vi "Parse Single Measurement.vi"(9 "Offset":i32, 10 "Measurement String":string) -> (1 "Measurement Metadata":T1, 2 "Measurement":dbl, 4 "Offset Past Token":i32)   [LabVIEW 2011, in "Keithley 2182.lvlib"]
doc: "Parses a single measurement into a numerical value and its corresponding metadata.\n\nAssumes all metadata is included in string, which includes:\n\n1. Reading\n2. Unit\n3. Channel\n\n[Mantissa][Exponent][Units], [Channel][Channel Units]\n\ne.g.\n-1.23456789E00VDC, 01INTCHAN"
uses:
  Keithley 2182.lvlib
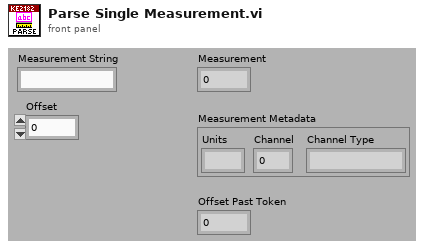
[diagram p1: front panel]
types:
  T1 = cluster{"Units":string, "Channel":i32, "Channel Type":string}
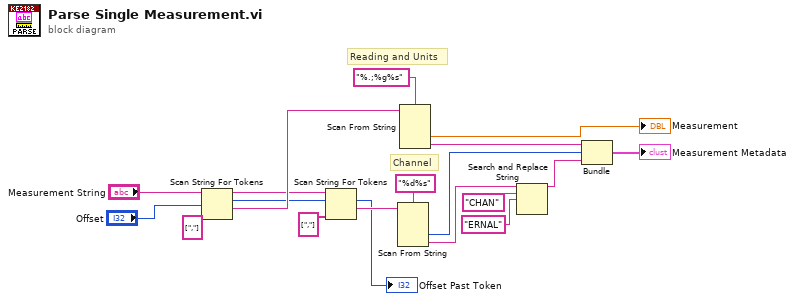
[diagram p0: block diagram]
diagram:
  # "Channel"
  # "Reading and Units"
  n1 = Scan String For Tokens(6:string[] [","] ("delimiters (\\s,\\t,\\r,\\n)"), 8:"Offset", 9:"Measurement String") -> (1:w17:string, 2:w14:i32, 3:w16:string)  [unwired: 3 in, 1 out]
  n2 = Scan String For Tokens(6:string[] [","] ("delimiters (\\s,\\t,\\r,\\n)"), 8:w14, 9:w16) -> (1:w12:string, 2:→"Offset Past Token":i32)  [unwired: 3 in, 2 out]
  n3 = Scan From String(format string="%d%s", input string=w12) -> (output 1=w11:i32, output 2=w10:string)  [unwired: 4 in, 3 out]
  n4 = Scan From String(format string="%.;%g%s", input string=w17) -> (output 1=→"Measurement":dbl, output 2=w13:string)  [unwired: 4 in, 3 out]
  n5 = Search and Replace String(input string=w10, search string="CHAN", replace string="ERNAL" ("replace string (\"\")")) -> (result string=w7:string)  [unwired: 5 in, 3 out]
  n6 = Bundle(w13, w11, "result string"=w7) -> (→"Measurement Metadata":cluster{string, i32, "result string":string})  [unwired: 1 in]
